vi "VI Test.vi"(6 "Aktion":T1, 8 "error in (no error)":errorcluster caption="Fehler (Eingang, kein Fehler)", 10 "Spülen":dbl=120.0, 11 "KommLoopTimer":u32) -> (0 "error out":errorcluster caption="Fehler (Ausgang)", 1 "Status Test":string, 2 "Fertig":bool, 3 "Referenz":sgl, 4 "Aktion":T1, 7 "Warten":dbl)   [LabVIEW 2020, in "EPA 1065.lvlib" / "HovaCAL Interference verificaton.lvlib"]
uses:
  HovaCAL Interference verificaton.lvlib
  Aktion Test.ctl
  Sprachverwaltung/FGV Aktion Tabelle zerlegen.ctl
  Aktion FGV Interference.ctl
  Aktion Index uebersetzten.ctl
  Seiten/CalGas Aufschaltung/FGV CalGas Aktionen.ctl
  Funktionstasten/Zustaende.ctl
  Funktionstasten/Funktionstasten-Aktion.ctl
  Seiten/CalGas Aufschaltung/Auswahl Aufschaltpunkt.ctl
  PNS/Aktionen FGV Grenzwerte.ctl
  Sprachverwaltung/Sprachverwaltung.lvlib
  Funktionstasten/Funktionstasten.lvlib
  Seiten/CalGas Aufschaltung/CalGas Aufschaltung.lvlib
  PNS/PNS.lvlib
  Linearisierung V2/Linearisierung v2.lvlib
  Linearisierung V2/Gasteiler/HovaCAL_Interface/Helper/Helper.lvlib
  Linearisierung V2/Gasteiler/HovaCAL_Interface/Kommunikation/Kommunikation.lvlib
  Linearisierung V2/Gasteiler/HovaCal/HovaCal.lvlib
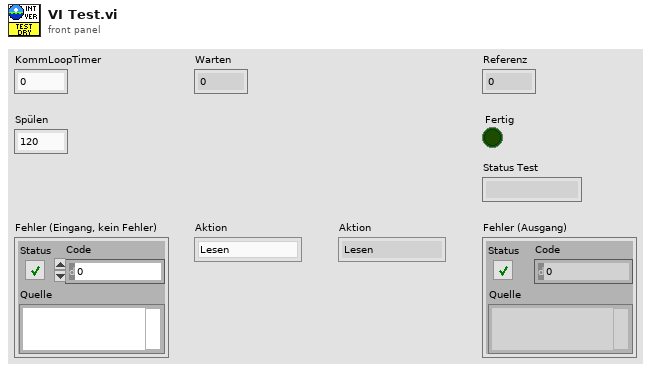
[diagram p1: front panel]
types:
  T1 = typedef "EPA 1065.lvlib/HovaCAL Interference verificaton.lvlib/Aktion Test.ctl" = enum16{"Lesen", "ini", "ini-Warten-Stabil", "Warten-Stabil", "ini-warten-aufzeichnen", "Warten-Aufzeichnen", "aufzeichnen", "fertig", "spülen", "abbrechen"}
  T2 = typedef "CalGas Aufschaltung.lvlib/FGV CalGas Aktionen.ctl" = enum16{"lesen", "Analysator Auswahl", "Def.CalGas", "Aufschaltung CalGas", "laden", "speichern", "KAL extrahieren"}
  T3 = typedef "EPA 1065.lvlib/HovaCAL Interference verificaton.lvlib/Aktion Index uebersetzten.ctl" = enum16{"lesen", "schreiben", "auswerten", "Referenzwert", "KompIndex", "RefInterferIndex", "KontrInterfIndex"}
  T4 = typedef "EPA 1065.lvlib/HovaCAL Interference verificaton.lvlib/Aktion FGV Interference.ctl" = enum16{"Lesen", "TestKonfig", "TestSetting", "Einheiten", "Ergebnis", "Laden", "Tabelle", "Speichern", "löschen"}
  T5 = typedef "Sprachverwaltung.lvlib/FGV Aktion Tabelle zerlegen.ctl" = enum16{"laden", "vereinzeln", "speichern"}
  T6 = typedef "Funktionstasten.lvlib/Funktionstasten-Aktion.ctl" = enum16{"Initialisieren", "Zustand setzen", "Taste gedrückt", "Fehler speichern", "Lesen", "Manuell", "Remote", "Bitparallel", "Samplepoint", "Zeit Prüfen", "reset Umschalten"}
  T7 = typedef "Funktionstasten.lvlib/Zustaende.ctl" = enum16{"Standby", "Pause", "Eco", "Messen", "Kalibrieren", "Spülen Filter", "Spülen Leitung", "Umgebungsluft", "0-Gas", "Cal-Gas", "CG zu PNS", "-------------", "Init 1", "Init 2", "Init 3", "Init 4", "Messen vorbereiten", "Messen durchführen", "Exit"}
  T8 = typedef "CalGas Aufschaltung.lvlib/Auswahl Aufschaltpunkt.ctl" = enum16{"über Filterblock", "Analysator direkt", "über PNS", "Entnahme", "Gasdivider"}
  T9 = typedef "PNS.lvlib/Aktionen FGV Grenzwerte.ctl" = enum16{"lesen", "Grenzw. schreiben", "Anweisungscode", "IP-Adresse", "laden", "speichern", "Anweisungscode vorgeben"}
  T10 = typedef "CalGas Aufschaltung.lvlib/Aufschaltung CalGas.ctl" = cluster{"Kalibriergas":T11, "Aufschaltpunkt":T8, "Analysator":T12}
  T11 = typedef "Auswahlfeld.ctl" = u16
  T12 = typedef "CalGas Aufschaltung.lvlib/Auswahl Analysator.ctl" = enum16{"FT-IR", "FID", "PMA", "PMA/FID/FT-IR"}
  T13 = typedef "EPA 1065.lvlib/HovaCAL Interference verificaton.lvlib/TestKonfig.ctl" = cluster{"TestKonfig H2O":T14, "TestKonfig Interferent":T20}
  T14 = typedef "EPA 1065.lvlib/HovaCAL Interference verificaton.lvlib/TestKonfig H2O.ctl" = cluster{"Modus":T15, "Komponente:":u16, "Eingangs Konzentration:":dbl, "Einheit":T16, "Anzahl Stufen":sgl, "Zeitdauer Stufen":sgl, "Max Fehler":sgl, "zusätzliche Zeitdauer Erster Punkt":sgl, "Punkte umkehren":bool, "Stufen Tabelle":T17, "HovaCAL Flow Input Cluster":T18, "HovaCAL Temperature":T19}
  T15 = typedef "EPA 1065.lvlib/HovaCAL Interference verificaton.lvlib/Modus.ctl" = u16
  T16 = typedef "Linearisierung v2.lvlib/SpanEinstellungen.lvlib/Einheit.ctl" = enum16{"ppm", "%"}
  T17 = typedef "Linearisierung v2.lvlib/Gasteiler.lvlib/Stufen Tabelle 10 Stufen.ctl" = string[][]
  T18 = typedef "Linearisierung v2.lvlib/Gasteiler.lvlib/HovaCAL_Interface.lvlib/Controls.lvlib/Flow Einstellung.ctl" = cluster{"HovaCAL Flow Input Cluster":dbl}
  T19 = typedef "Linearisierung v2.lvlib/Gasteiler.lvlib/HovaCAL_Interface.lvlib/Controls.lvlib/Temp Sollwerte Anzeige.ctl" = dbl[]
  T20 = typedef "EPA 1065.lvlib/HovaCAL Interference verificaton.lvlib/TestKonfig Interferents.ctl" = cluster{"MFC1":enum16{"MFC 1"}, "Eingangs Konzentration MFC1":dbl, "Einheit MFC1 Eingang":T16, "Ausgangs Konzentration MFC1":dbl, "Einheit MFC1 Ausgang":T16, "MFC2":T21, "Referenz-Interferent:":u16, "Gasflaschen Nr MFC2":string, "Accuracy MFC2":string, "Eingangs Konzentration MFC2":dbl, "Einheit MFC2 Eingang":T16, "Ausgangs Konzentration MFC2":dbl, "Einheit MFC2 Ausgang":T16, "MFC3":T21, "Kontroll-Interferent:":u16, "Gasflaschen Nr MFC3":string, "Accuracy MFC3":string, "Eingangs Konzentration MFC3":dbl, "Einheit MFC3 Eingang":T16, "Ausgangs Konzentration MFC3":dbl, "Einheit MFC3 Ausgang":T16, "Gasflasche MFC2":T22, "Gasflasche MFC3":T22}
  T21 = typedef "EPA 1065.lvlib/HovaCAL Interference verificaton.lvlib/MFCAuswahl.ctl" = u16
  T22 = typedef "System Einstellungen V2.lvlib/Gasflasche Auswahl.ctl" = u16
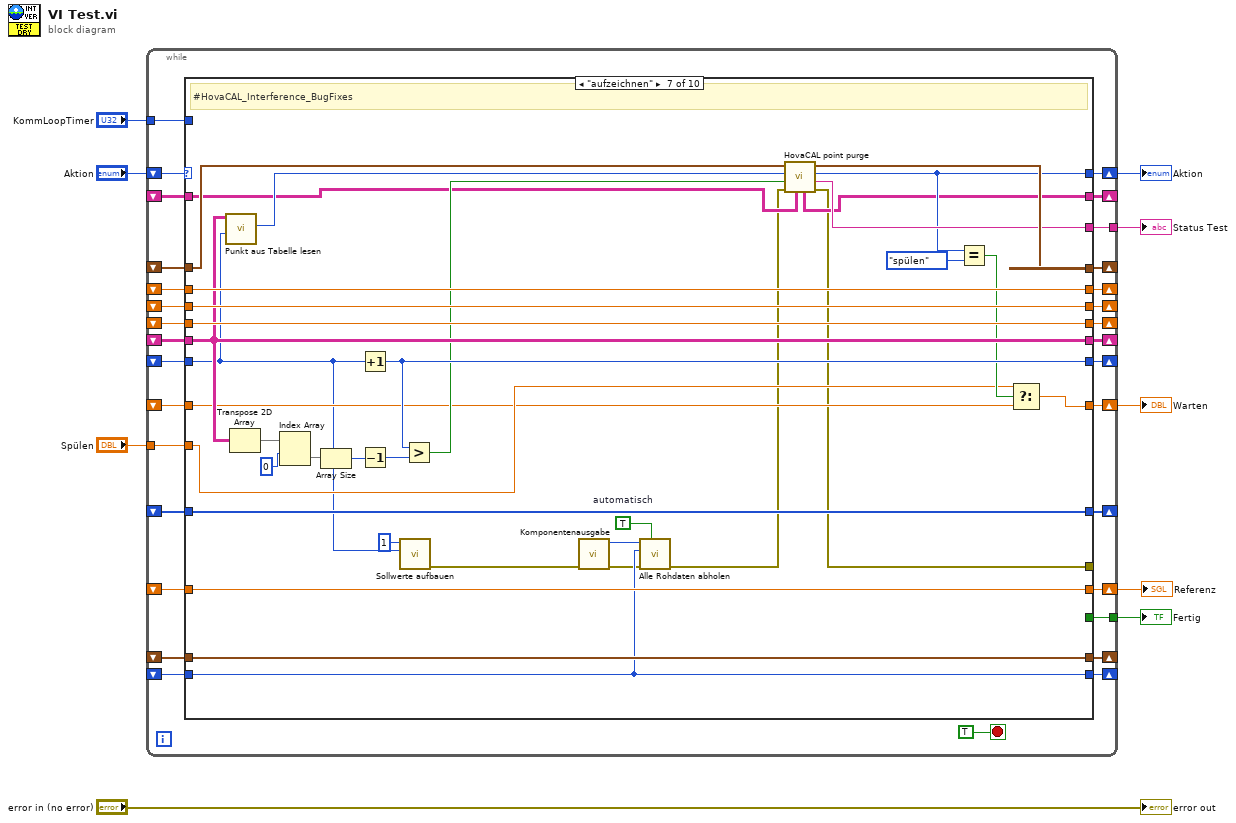
[diagram p0: block diagram]
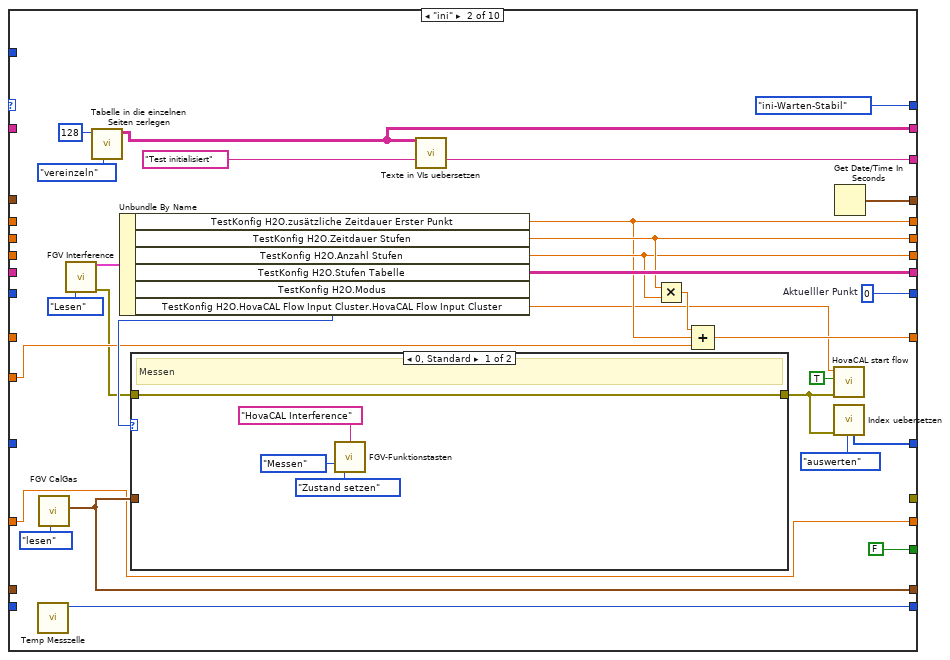
[diagram p3: hidden frame]
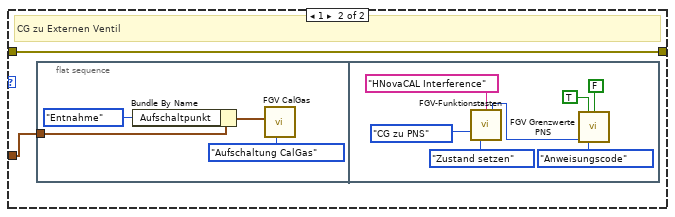
[diagram p4: hidden frame]
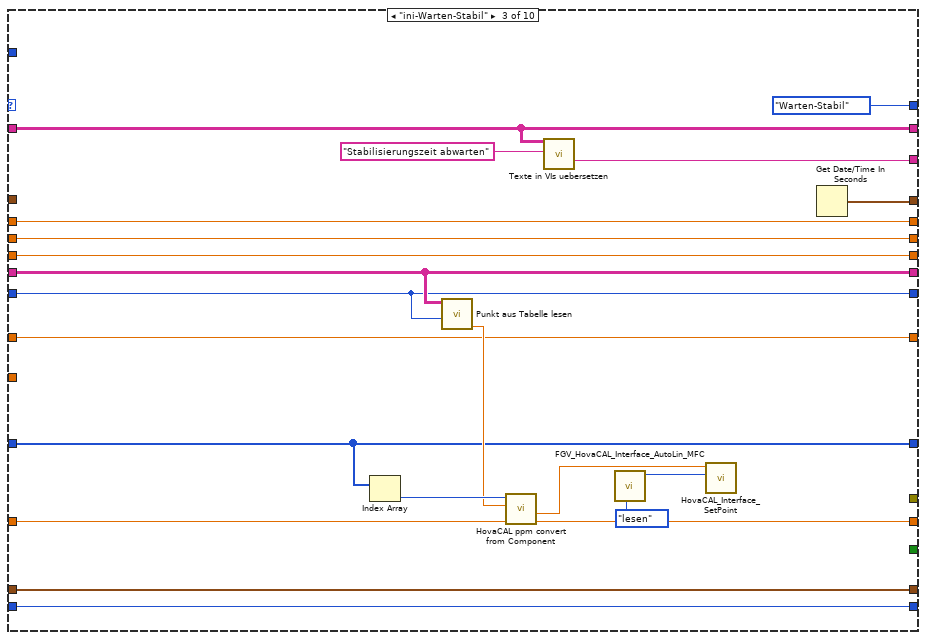
[diagram p5: hidden frame]
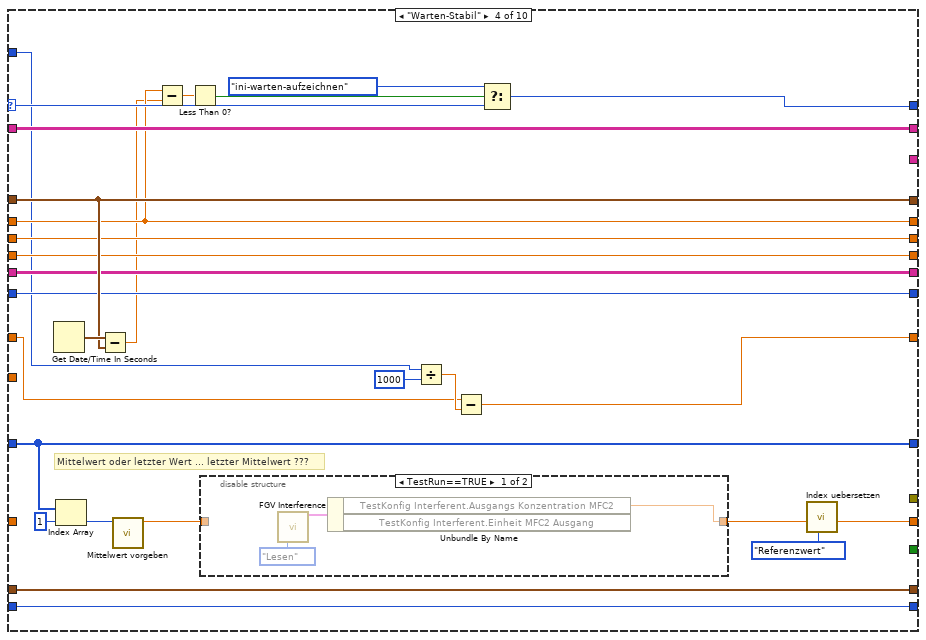
[diagram p6: hidden frame]
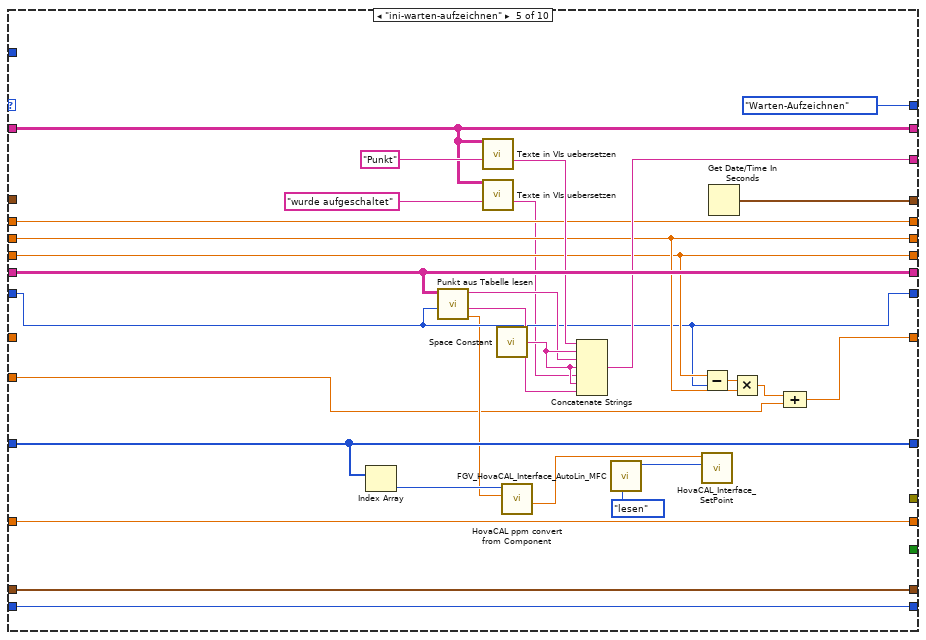
[diagram p8: hidden frame]
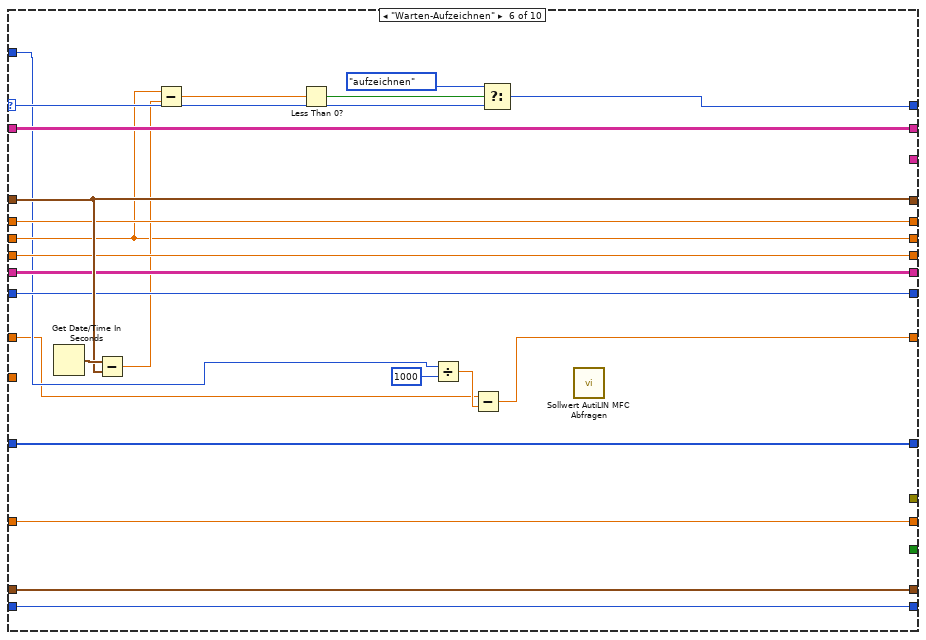
[diagram p9: hidden frame]
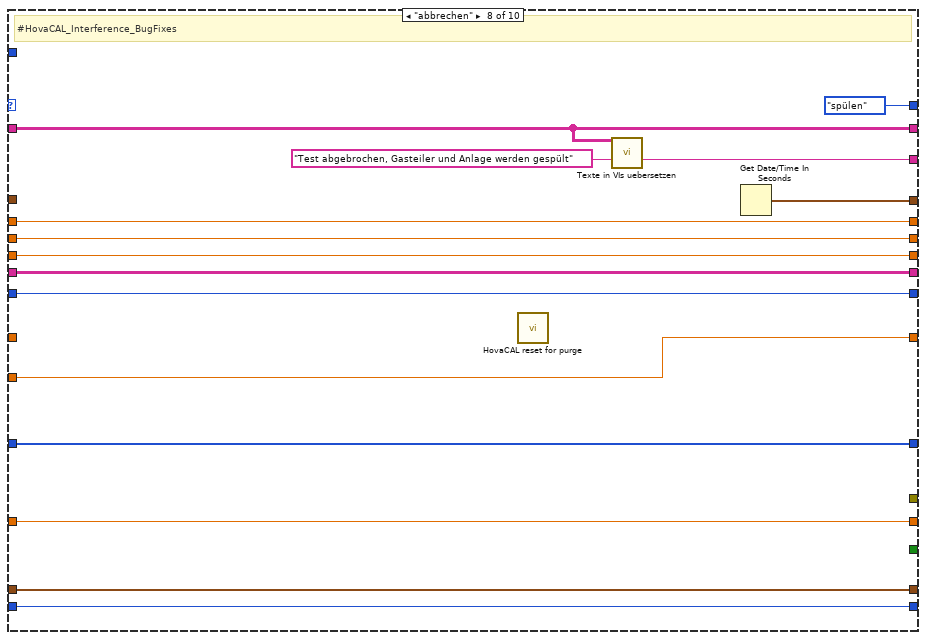
[diagram p10: hidden frame]
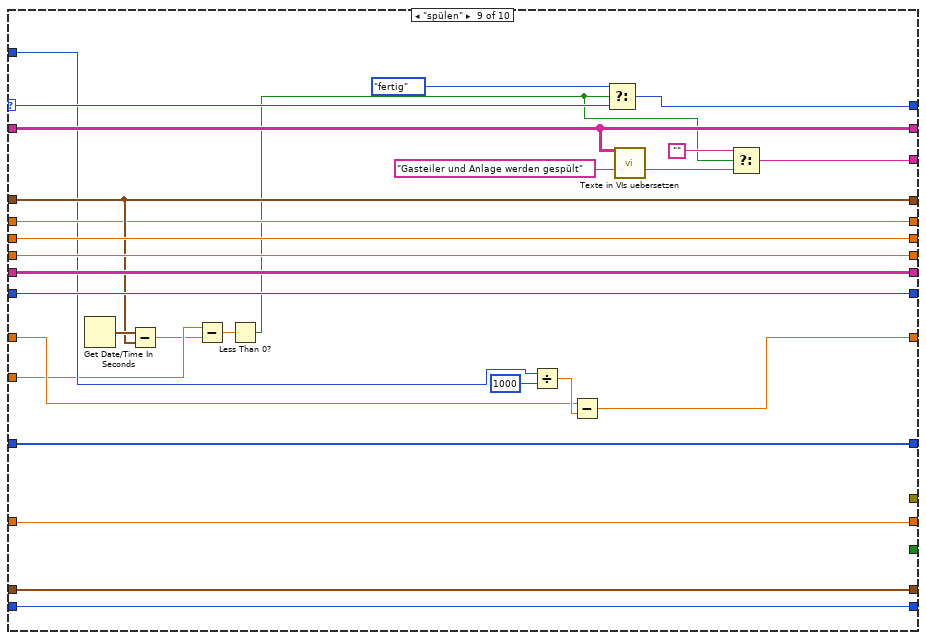
[diagram p11: hidden frame]
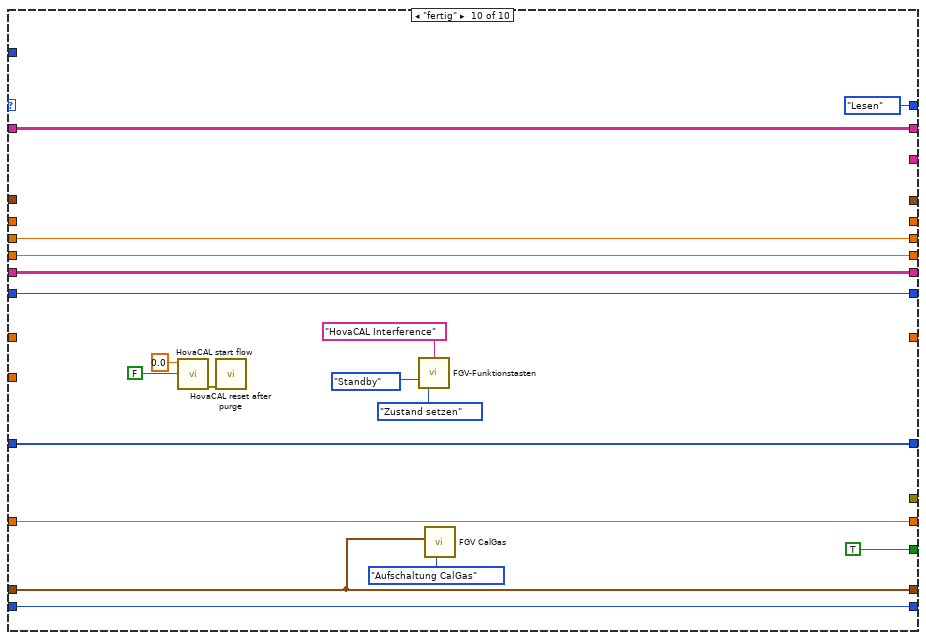
[diagram p12: hidden frame]
diagram:
  n1 = while {
    shift-right: [w39] -> _
    shift-left: _ -> [w38]
    tunnel: [w37] -> w8
    shift-right: [w36] -> _
    shift-left: _ -> [w35]
    shift-right: [w34] -> _
    shift-left: _ -> [w33]
    shift-right: [w32] -> _
    shift-left: _ -> [w31]
    shift-right: [w29] -> w6
    shift-left: "Aktion" -> [w30]
    tunnel: [w28] -> w5
    shift-right: [w26] -> _
    shift-left: _ -> [w25]
    shift-right: [w24] -> w3
    shift-left: _ -> [w23]
    shift-right: [w22] -> _
    shift-left: _ -> [w21]
    shift-right: [w20] -> _
    shift-left: _ -> [w19]
    shift-right: [w18] -> _
    shift-left: _ -> [w17]
    tunnel: "Spülen" -> [w16]
    shift-right: [w27] -> w4
    shift-left: _ -> [w15]
    shift-right: [w14] -> _
    shift-left: _ -> [w13]
    shift-right: [w12] -> _
    shift-left: _ -> [w11]
    tunnel: "KommLoopTimer" -> [w10]
    stop <- TRUE stop-if-true
    n2 = case shown="\"aufzeichnen\"" w30 {
      selector: w30 -> [w48 _ _ w141 _ w197 _ _ w269 _]
      tunnel: [w51 w80 w117 w144 w154 w200 w222 w237 w271 _] -> w39
      tunnel: w38 -> [w51 _ _ w144 _ w200 w223 _ w271 _]
      tunnel: [_ w77 w116 _ w168 _ w221 w238 w257 _] -> w37
      tunnel: [w50 w76 w114 w140 w153 w196 w204 w239 w265 w297] -> w36
      tunnel: w35 -> [w50 _ w114 w140 w153 w196 w205 w239 w265 w297]
      tunnel: [w49 w53 w103 w119 w167 w192 w224 w241 w279 w295] -> w34
      tunnel: w33 -> [w49 _ w103 w119 w167 w192 w224 w241 w279 w295]
      tunnel: [_ w61 w112 w132 w161 w194 w236 w244 w270 _] -> w32
      tunnel: w31 -> [_ _ w112 w132 w161 w194 w236 w244 w270 _]
      tunnel: [w48 Aktion_Test."ini-Warten-Stabil" ("Enum") Aktion_Test."Warten-Stabil" ("Enum") w139 Aktion_Test."Warten-Aufzeichnen" ("Enum") w195 w216 Aktion_Test."spülen" ("Aktion") w268 Aktion_Test."Lesen" ("Aktion")] -> w29
      tunnel: [_ FALSE ("Erreicht") _ _ _ _ _ _ _ TRUE] -> w28
      tunnel: [_ w60 w98 w125 w160 w180 w211 w243 w260 _] -> w27
      tunnel: [w47 w68 w111 w138 w176 w193 w235 w251 w278 w290] -> w26
      tunnel: w25 -> [w47 _ w111 w138 w176 w193 w235 w251 w278 w290]
      tunnel: [w46 w66 w110 w118 w175 w179 w234 w250 w277 w289] -> w24
      tunnel: w23 -> [w46 w66 w110 _ w175 w179 w234 w250 w277 w289]
      tunnel: [w45 w63 w109 w137 w164 w186 w233 w249 w276 w288] -> w22
      tunnel: w21 -> [w45 _ w109 w137 w164 w186 w233 w249 w276 w288]
      tunnel: [w44 w62 w108 w136 w163 w191 w232 w248 w275 w287] -> w20
      tunnel: w19 -> [w44 _ w108 w136 w163 w191 w232 w248 w275 w287]
      tunnel: [w43 w65 w102 w135 w173 w190 w226 w247 w274 w286] -> w18
      tunnel: w17 -> [w43 _ w102 w135 w173 w190 w226 w247 w274 w286]
      tunnel: w16 -> [_ w59 _ _ w150 _ w213 w243 w255 _]
      tunnel: w15 -> [_ _ w98 w126 _ w181 w212 _ w259 _]
      tunnel: [w42 w58 w101 w134 w162 w189 w225 w246 w273 w285] -> w14
      tunnel: w13 -> [w42 _ w101 w134 w162 w189 w210 w246 w273 w285]
      tunnel: [w41 w54 w99 w130 w151 w185 w217 w245 w264 w282] -> w12
      tunnel: w11 -> [w41 _ w99 w130 w151 w185 w217 w245 w264 w282]
      tunnel: [_ _ _ _ _ _ w202 _ _ _] -> _
      tunnel: w10 -> [_ _ _ w127 _ w182 _ _ w261 _]
      frame "Lesen", Default {
      }
      frame "ini" {
        w58 = 0  # Aktuelller Punkt
        n3 = call "Temp Messzelle.vi"() -> ("Temp. Messzelle"=w54:i32)  [unwired: 11 in]
        n4 = call "FGV CalGas.vi"("Aktionen"=FGV_CalGas_Aktionen."lesen") -> ("Aufschaltung CalGas"=w68:T10)  [unwired: 6 in, 4 out]
        n5 = call "FGV Interference.vi"("Aktion FGV Interference"=Aktion_FGV_Interference."Lesen") -> ("TestKonfig"=w73:T13, "error out"=w57:errorcluster)  [unwired: 9 in, 4 out]
        n6 = call "Tabelle in die einzelnen Seiten zerlegen.vi"("Aktion"=FGV_Aktion_Tabelle_zerlegen."vereinzeln", "Index (Seite)"=128) -> ("Sprachliste"=w76:string[][])  [unwired: 7 in, 2 out]
        n7 = Unbundle By Name(w73) -> ("TestKonfig H2O.zusätzliche Zeitdauer Erster Punkt"=w61:sgl, "TestKonfig H2O.Zeitdauer Stufen"=w63:sgl, "TestKonfig H2O.Anzahl Stufen"=w62:sgl, "TestKonfig H2O.Stufen Tabelle"=w65:T17, "TestKonfig H2O.Modus"=w67:T15, "TestKonfig H2O.HovaCAL Flow Input Cluster.HovaCAL Flow Input Cluster"=w52:dbl)
        n8 = case shown="0, Standard" w67 {
          tunnel: w68 -> [_ w86]
          tunnel: [w81 w85] -> w56
          tunnel: w57 -> [w81 w85]
          frame 0, Default {
            # "Messen"
            n9 = call "FGV-Funktionstasten.vi"("Herkunft"="HovaCAL Interference", "Zustand"=Zustaende."Messen", "Aktion"=Funktionstasten-Aktion."Zustand setzen") -> ()  [unwired: 5 in, 8 out]
          }
          frame 1 {
            # "CG zu Externen Ventil"
            n10 = flat-sequence {
              tunnel: w86 -> [w89]
              frame #0 {
                n11 = Bundle By Name(cluster=w89, "Aufschaltpunkt"=Auswahl_Aufschaltpunkt."Entnahme") -> (w90:T10)
                n12 = call "FGV CalGas.vi"("Aktionen"=FGV_CalGas_Aktionen."Aufschaltung CalGas", "Aufschaltung CalGas"=w90) -> ()  [unwired: 5 in, 5 out]
              }
              frame #1 {
                n13 = call "FGV-Funktionstasten.vi"("Herkunft"="HNovaCAL Interference", "Zustand"=Zustaende."CG zu PNS", "Aktion"=Funktionstasten-Aktion."Zustand setzen") -> ("Samplepoint"=w91:u16)  [unwired: 5 in, 7 out]
                n14 = call "FGV Grenzwerte PNS.vi"("T90"=TRUE ("T90 lüften"), "T90 lüften"=FALSE, "Samplepoint"=w91, "Aktionen FGV Grenzwerte"=Aktionen_FGV_Grenzwerte."Anweisungscode") -> ()  [unwired: 9 in, 3 out]
              }
            }
          }
        }
        n15 = call "Texte in VIs uebersetzen.vi"("Sprachliste"=w76, "String zum Übersetzen"="Test initialisiert") -> ("String zum Übersetzen"=w77:string)  [unwired: 9 in, 4 out]
        n16 = Multiply(x=w63, y=w62) -> (x*y=w64:sgl)
        n17 = Compound Arithmetic op=ADD(w64, w61, w59) -> (w60:dbl)
        n18 = call "HovaCAL start flow.vi"("error in (no error)"=w56, "run"=TRUE, "total flow setpoint"=w52) -> ()  [unwired: 8 in, 1 out]
        n19 = call "Index uebersetzen.vi"("Aktion"=Aktion_Index_uebersetzten."auswerten", "error in (no error)"=w56) -> ("Komponenten Indices"=w53:i32[])  [unwired: 4 in, 5 out]
        n20 = Get Date/Time In Seconds() -> (seconds since 1Jan1904=w80:timestamp)
      }
      frame "ini-Warten-Stabil" {
        n21 = Index Array(array=w103) -> (element=w107:i32)  [unwired: 1 in]
        n22 = call "Punkt aus Tabelle lesen.vi"("Index"=w101, "Stufen Tabelle"=w102) -> ("Sollwert"=w106:sgl)  [unwired: 6 in, 3 out]
        n23 = call "HovaCAL ppm convert from Component.vi"("Konzentration"=w106, "Gasnummer"=w107) -> ("Konzentration in ppm"=w104:dbl)  [unwired: 5 in, 4 out]
        n24 = call "Texte in VIs uebersetzen.vi"("Sprachliste"=w114, "String zum Übersetzen"="Stabilisierungszeit abwarten") -> ("String zum Übersetzen"=w116:string)  [unwired: 9 in, 4 out]
        n25 = call "FGV_HovaCAL_Interface_AutoLin_MFC.vi"("Aktion"=enum16{"lesen", "schreiben"}."lesen") -> ("AutoLin MFC out"=w105:u16)  [unwired: 7 in, 3 out]
        n26 = call "HovaCAL_Interface_SetPoint.vi"("AutoLin MFC Index"=w105, "Konzentration"=w104) -> ()  [unwired: 9 in, 1 out]
        n27 = Get Date/Time In Seconds() -> (seconds since 1Jan1904=w117:timestamp)
      }
      frame "Warten-Stabil" {
        # "Mittelwert oder letzter Wert ... letzter Mittelwert ???"
        n28 = Get Date/Time In Seconds() -> (seconds since 1Jan1904=w145:timestamp)
        n29 = Index Array(array=w119, index=1 ("Index")) -> (element=w123:i32)
        n30 = Subtract(x=w145, y=w144) -> (x-y=w131:dbl)
        n31 = call "Mittelwert vorgeben.vi"("Komponente"=w123) -> ("Mittelwert"=w121:sgl)  [unwired: 10 in]
        n32 = Subtract(x=w132, y=w131) -> (x-y=w133:dbl)
        n33 = Less Than 0?(x=w133) -> (x < 0?=w142:bool)
        n34 = disable-structure shown="TestRun==TRUE" {
          disable-tunnel: w121 -> [_ w149]
          disable-tunnel: [w146 w149] -> w120
          frame condition #0 {
            n35 = call "FGV Interference.vi"("Aktion FGV Interference"=Aktion_FGV_Interference."Lesen") -> ("TestKonfig"=w148:T13)  [unwired: 9 in, 5 out]
            n36 = Unbundle By Name(w148) -> ("TestKonfig Interferent.Ausgangs Konzentration MFC2"=w146:dbl)  [unwired: 1 out]
          }
          frame condition #1 (active) {
          }
        }
        n37 = Divide(x=w127, y=u32 1000) -> (x/y=w128:dbl)
        n38 = Subtract(x=w126, y=w128) -> (x-y=w125:dbl)
        n39 = Select(t=Aktion_Test."ini-warten-aufzeichnen" ("Enum"), s=w142, f=w141) -> (s? t:f=w139:T1)
        n40 = call "Index uebersetzen.vi"("Aktion"=Aktion_Index_uebersetzten."Referenzwert", "Referenz in"=w120) -> ("Referenz out"=w118:sgl)  [unwired: 4 in, 5 out]
      }
      frame "ini-warten-aufzeichnen" {
        n41 = Index Array(array=w167) -> (element=w159:i32)  [unwired: 1 in]
        n42 = call "Punkt aus Tabelle lesen.vi"("Index"=w162, "Stufen Tabelle"=w173) -> (0:"Sollwert"=w158:sgl, 1:"Sollwert"=w169:string, "Punkt"=w170:string)  [unwired: 6 in, 1 out]
        n43 = call "Texte in VIs uebersetzen.vi"("Sprachliste"=w153, "String zum Übersetzen"="Punkt") -> ("String zum Übersetzen"=w171:string)  [unwired: 9 in, 4 out]
        n44 = call "Texte in VIs uebersetzen.vi"("Sprachliste"=w153, "String zum Übersetzen"="wurde aufgeschaltet" ("String")) -> ("String zum Übersetzen"=w152:string)  [unwired: 9 in, 4 out]
        n45 = call <vilib>:"Space Constant.vi"() -> ("String"=w172:string)
        n46 = call "HovaCAL ppm convert from Component.vi"("Konzentration"=w158, "Gasnummer"=w159) -> ("Konzentration in ppm"=w155:dbl)  [unwired: 5 in, 4 out]
        n47 = Concatenate Strings(w171, w172, w170, w172, w152, w172, w169) -> (w168:string)
        n48 = call "FGV_HovaCAL_Interface_AutoLin_MFC.vi"("Aktion"=enum16{"lesen", "schreiben"}."lesen") -> ("AutoLin MFC out"=w156:u16)  [unwired: 7 in, 3 out]
        n49 = Subtract(x=w163, y=w162) -> (x-y=w165:sgl)
        n50 = call "HovaCAL_Interface_SetPoint.vi"("AutoLin MFC Index"=w156, "Konzentration"=w155) -> ()  [unwired: 9 in, 1 out]
        n51 = Get Date/Time In Seconds() -> (seconds since 1Jan1904=w154:timestamp)
        n52 = Multiply(x=w165, y=w164) -> (x*y=w166:sgl)
        n53 = Compound Arithmetic op=ADD(w166, w150) -> (w160:dbl)
      }
      frame "Warten-Aufzeichnen" {
        n54 = Get Date/Time In Seconds() -> (seconds since 1Jan1904=w201:timestamp)
        n55 = Subtract(x=w201, y=w200) -> (x-y=w187:dbl)
        n56 = Subtract(x=w186, y=w187) -> (x-y=w188:dbl)
        n57 = Less Than 0?(x=w188) -> (x < 0?=w198:bool)
        n58 = Divide(x=w182, y=u32 1000) -> (x/y=w183:dbl)
        n59 = Subtract(x=w181, y=w183) -> (x-y=w180:dbl)
        n60 = Select(t=Aktion_Test."aufzeichnen" ("Enum"), s=w198, f=w197) -> (s? t:f=w195:T1)
        n61 = call "Sollwert AutiLIN MFC Abfragen.vi"() -> ()  [unwired: 12 in]
      }
      frame "aufzeichnen" {
        w208 = TRUE  # automatisch
        # "#HovaCAL_Interference_BugFixes"
        n62 = call "Punkt aus Tabelle lesen.vi"("Index"=w210, "Stufen Tabelle"=w226) -> ("Punkt"=w220:i32)  [unwired: 6 in, 3 out]
        n63 = Transpose 2D Array(2D array=w226) -> (transposed array=w228:T17)
        n64 = Index Array(array=w228, index (row)=0 ("Index (Zeile)")) -> (element=w229:string[])  [unwired: 1 in]
        n65 = Array Size(array=w229) -> (size(s)=w230:i32)
        n66 = Increment(x=w210) -> (x+1=w225:i32)
        n67 = Decrement(x=w230) -> (x-1=w227:i32)
        n68 = call "Sollwerte aufbauen.vi"("Punkt"=w210, "Aktuelle Gasnummer"=u8 1) -> ("error out"=w218:errorcluster)  [unwired: 9 in]
        n69 = Greater?(x=w225, y=w227) -> (0:w219:bool)
        n70 = call "Komponentenausgabe.vi"("error in (no error)"=w218) -> ("error out"=w209:errorcluster, "Gaskomponente"=w207:T11)  [unwired: 7 in, 2 out]
        n71 = call "Alle Rohdaten abholen.vi"("automatisch"=w208, "error in (no error)"=w209, "Temp. Messzelle G-nr."=w217, "Gasindex"=w207) -> ("error out"=w203:errorcluster)  [unwired: 6 in, 1 out]
        n72 = call "HovaCAL point purge.vi"("Sprachliste"=w205, "error in (no error)"=w203, "letzter Punkt"=w219, "Punkt"=w220, "Timer (Eingang)"=w223) -> ("error out"=w202:errorcluster, "Status"=w221:string, "Aktion out"=w216:T1, "Timer (Ausgang)"=w222:timestamp, "Sprachliste out"=w204:string[][])  [unwired: 2 in]
        n73 = Equal?(x=w216, y=Aktion_Test."spülen") -> (x = y?=w214:bool)
        n74 = Select(t=w213, s=w214, f=w212) -> (s? t:f=w211:dbl)
      }
      frame "abbrechen" {
        # "#HovaCAL_Interference_BugFixes"
        n75 = call "HovaCAL reset for purge.vi"() -> ()  [unwired: 11 in, 1 out]
        n76 = call "Texte in VIs uebersetzen.vi"("Sprachliste"=w239, "String zum Übersetzen"="Test abgebrochen, Gasteiler und Anlage werden gespült" ("String 2 hinzufügen")) -> ("String zum Übersetzen"=w238:string)  [unwired: 9 in, 4 out]
        n77 = Get Date/Time In Seconds() -> (seconds since 1Jan1904=w237:timestamp)
      }
      frame "spülen" {
        n78 = Get Date/Time In Seconds() -> (seconds since 1Jan1904=w272:timestamp)
        n79 = Subtract(x=w272, y=w271) -> (x-y=w254:dbl)
        n80 = Subtract(x=w255, y=w254) -> (x-y=w253:dbl)
        n81 = Less Than 0?(x=w253) -> (x < 0?=w252:bool)
        n82 = Divide(x=w261, y=u32 1000) -> (x/y=w262:dbl)
        n83 = Subtract(x=w259, y=w262) -> (x-y=w260:dbl)
        n84 = Select(t=Aktion_Test."fertig" ("Aktion"), s=w252, f=w269) -> (s? t:f=w268:T1)
        n85 = call "Texte in VIs uebersetzen.vi"("Sprachliste"=w265, "String zum Übersetzen"="Gasteiler und Anlage werden gespült" ("String 2 hinzufügen")) -> ("String zum Übersetzen"=w258:string)  [unwired: 9 in, 4 out]
        n86 = Select(t="", s=w252, f=w258) -> (s? t:f=w257:string)
      }
      frame "fertig" {
        n87 = call "HovaCAL start flow.vi"("run"=FALSE, "total flow setpoint"=0.0) -> ("error out"=w280:errorcluster)  [unwired: 9 in]
        n88 = call "HovaCAL reset after purge.vi"("Fehler (Eingang, kein Fehler)"=w280) -> ()  [unwired: 10 in, 1 out]
        n89 = call "FGV-Funktionstasten.vi"("Herkunft"="HovaCAL Interference", "Zustand"=Zustaende."Standby", "Aktion"=Funktionstasten-Aktion."Zustand setzen") -> ()  [unwired: 5 in, 8 out]
        n90 = call "FGV CalGas.vi"("Aktionen"=FGV_CalGas_Aktionen."Aufschaltung CalGas", "Aufschaltung CalGas"=w290) -> ()  [unwired: 5 in, 5 out]
      }
    }
  }
  "Status Test" <- w8
  "Warten" <- w4
  "Aktion" <- w6
  "Fertig" <- w5
  "Referenz" <- w3
  "error out" <- "error in (no error)"
